vi "PID Autotuning Design (Auto).vi"(5 "Ziegler-Nichols Speed":u16(ring) items=["Fast", "Normal", "Slow"], 6 "Controller Gain (K)":dbl, 7 "Type of Controller":u16(ring) items=["P", "PI", "PID"], 8 "dt (s)":dbl, 9 "closed-loop?":bool, 10 "Response signal":dbl[](array[numeric]), 11 "Stimulus signal":dbl[](array[numeric])) -> (1 "PID gains":T2, 2 "response operating point":dbl, 3 "stimulus operating point":dbl, 4 "Plant Parameters":T1)   [LabVIEW 2020, in "NI_PID_autopid.lvlib"]
doc: "Implements autotuning using the tuning method associated with the polymorphic instance you select. This VI generates PID parameters based on the <B>Stimulus signal</B> and <B>Response signal</B> you specify. You can use this VI to generate initial parameters when you do not have sufficient information about the system you want to tune. You must manually select the polymorphic instance to use."
uses:
  <vilib>/addons/control/pid/NI_PID_autopid.lvlib
  <vilib>/addons/control/pid/NI_PID_pid.lvlib
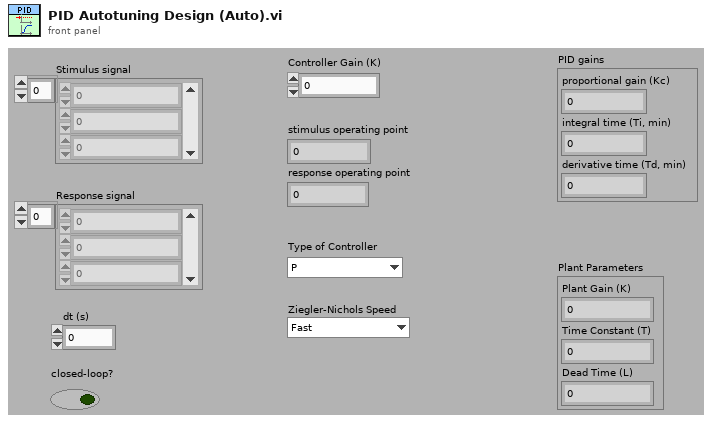
[diagram p1: front panel]
types:
  T1 = cluster{"Plant Gain (K)":dbl, "Time Constant (T)":dbl, "Dead Time (L)":dbl}
  T2 = cluster{"proportional gain (Kc)":dbl, "integral time (Ti, min)":dbl, "derivative time (Td, min)":dbl}
  T3 = enum16{"Academic (Standard)", "Parallel", "Series"}
  T4 = cluster{"OL Gain (Kp)":dbl, "OL Time Constant (T)":dbl, "Dead Time (L) Out":dbl}
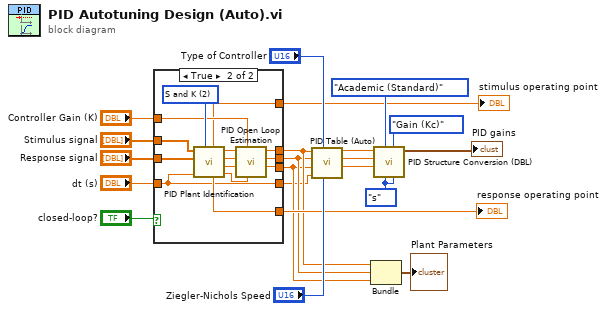
[diagram p0: block diagram]
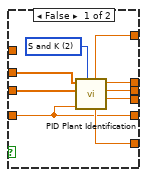
[diagram p2: hidden frame]
diagram:
  w14 = enum16{"min", "s"}."s" ("Integral Unit")
  n1 = case shown="True" "closed-loop?" {
    tunnel: "Response signal" -> [w29 w42]
    tunnel: "Stimulus signal" -> [w28 w43]
    tunnel: [w27 w34] -> w10
    tunnel: [w26 w33] -> w9
    tunnel: [w25 w40] -> w8
    tunnel: [w24 w41] -> w7
    tunnel: [w23 w32] -> w6
    tunnel: "dt (s)" -> [w22 w31]
    tunnel: "Controller Gain (K)" -> [_ w35]
    tunnel: [w22 w31] -> w1
    frame False {
      w30 = u16 2 items=["Z-N", "First Order", "S and K"] ("Ring")
      n2 = call <vilib>:"PID Plant Identification.vi"("Method"=w30, "Sampling Time"=w22, "Response signal"=w29, "Stimulus signal"=w28) -> ("Dead Time (L)"=w23:dbl, "Time Constant (T)"=w24:dbl, "Plant Gain (K)"=w25:dbl, "response offset"=w26:dbl, "stimulus offset"=w27:dbl)  [unwired: 1 in, 2 out]
    }
    frame True {
      w44 = u16 2 items=["Z-N", "First Order", "S and K", "Second Order"] ("Method")
      n3 = call <vilib>:"PID Plant Identification.vi"("Method"=w44, "Sampling Time"=w31, "Response signal"=w42, "Stimulus signal"=w43) -> ("Time Constant (T) 2"=w36:dbl, "Dead Time (L)"=w37:dbl, "Time Constant (T)"=w38:dbl, "Plant Gain (K)"=w39:dbl, "response offset"=w33:dbl, "stimulus offset"=w34:dbl)  [unwired: 1 in, 1 out]
      n4 = call <vilib>:"PID Open Loop Estimation.vi"("CL Time Constant (T) 2"=w36, "Controller Gain (K)"=w35, "Dead Time (L)"=w37, "CL Time Constant (Tcl)"=w38, "CL Gain (Kcl)"=w39) -> ("Dead Time (L) Out"=w32:dbl, "OL Time Constant (T)"=w41:dbl, "OL Gain (Kp)"=w40:dbl)  [unwired: 4 in]
    }
  }
  "stimulus operating point" <- w10
  "response operating point" <- w9
  n5 = call <vilib>:"PID Table (Auto).vi"("Ziegler-Nichlos Speed"="Ziegler-Nichols Speed", "Type of Controller"="Type of Controller", "dT"=w1, "Dead Time (L)"=w6, "Time Constant (T)"=w7, "Plant Gain (K)"=w8) -> ("Derivative Time (Td)"=w17:dbl, "Integral Time (Ti)"=w18:dbl, "Proportional Gain (Kp)"=w19:dbl)  [unwired: 3 in]
  n6 = Bundle("OL Gain (Kp)"=w8, "OL Time Constant (T)"=w7, "Dead Time (L) Out"=w6) -> (→"Plant Parameters":T4)  [unwired: 1 in]
  n7 = call <vilib>:"PID Structure Conversion (DBL).vi"("derivative unit"=w14, "proportional unit"=enum16{"Gain (Kc)", "Band (PB)"}."Gain (Kc)" ("Proportional Unit"), "integral unit"=w14, "PID structure"=T3."Academic (Standard)" ("PID Structure"), "derivative"=w17, "integral"=w18, "proportional"=w19) -> ("PID gains"=→"PID gains":T2)  [unwired: 4 in]
